vi "http read response.vi"(8 "error in (no error)":errorcluster, 9 "buf_len":i32, 10 "buf_ptr":string, 11 "handle":u64) -> (0 "error out":errorcluster, 1 "function return":i32, 2 "buf_ptr out":string, 3 "handle out":u64)   [LabVIEW 2020, in "reqwest-labview.lvlib"]
doc: "int http_read_response(void *handle,\n unsigned char *buf_ptr,\n int buf_len);"
uses:
  reqwest-labview.lvlib
  lib_reqwest_labview_64.dll
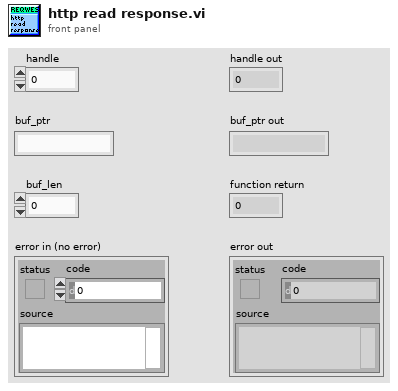
[diagram p1: front panel]
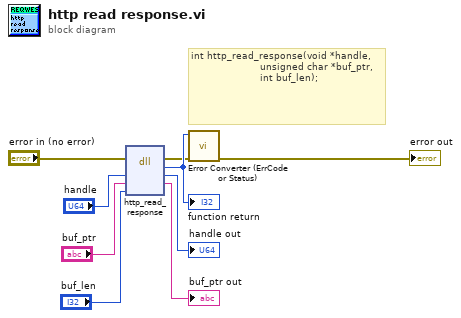
[diagram p0: block diagram]
diagram:
  # "int http_read_response(void *handle,\n                       unsigned char *buf_ptr,\n                       int buf_len);"
  n1 = dll-call lib="C:/code/reqwest-labview/lv-src/shared-library/lib_reqwest_labview_*.*" fn="http_read_response"(error in="error in (no error)", "handle"="handle", "buf_ptr"="buf_ptr", "buf_len"="buf_len") -> (error out=w2:errorcluster, "return type"=w9:i32, "handle"=→"handle out":u64, "buf_ptr"=→"buf_ptr out":string)  [unwired: 3 in, 1 out]
  "function return" <- w9
  n2 = call "Error Converter (ErrCode or Status).vi"("error in (no error)"=w2, "error code"=w9) -> ("error out"=→"error out":errorcluster)  [unwired: 9 in]
